vi "Single Button Toggle.vi"(1 "Input":bool) -> (0 "Output":bool)   [LabVIEW 2012]
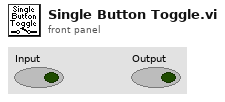
[diagram p1: front panel]
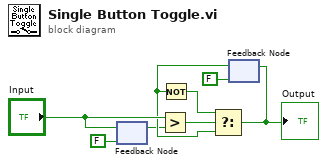
[diagram p0: block diagram]
diagram:
  n1 = feedback #1(FALSE ("L Drive Button 5")) -> (w1:bool)
  n2 = feedback-in #1("Input") -> ()
  n3 = Greater?(x="Input", y=w1) -> (0:w3:bool)
  n4 = feedback #2(FALSE) -> (w5:bool)
  n5 = Not(x=w5) -> (.not. x?=w4:bool)
  n6 = Select(t=w4, s=w3, f=w5) -> (s? t:f=w8:bool)
  "Output" <- w8
  n7 = feedback-in #2(w8) -> ()
